vi "CCD1字符识别定位核心转换.vi"(0 "Image In":T1, 1 "ROI Descriptor":T3={"Global Rectangle"=[566, 503, 2033, 1507], "Contours"=[{"ID"=enum."External", "Type"=3, "Coordinates"=[566, 503, 2033, 1507]}]} {"Contours"."Type" items=["No Selection", "Point", "Line", "Rectangle", "Oval", "Polygon", "Freehand Region", "Annulus", "Unused2", "Unused3", "Broken Line", "Freehand Line", "Rotated Rectangle"]}, 2 "Settings":T6={"Curve Parameters"={"Extraction Mode"=0, "Edge Threshold"=35, "Edge Filter Size"=1, "Min Length"=25, "Row Search Step Size"=15, "Col Search Step Size"=15, "Max Endpoint Gap"=10, "Closed"=FALSE, "Subpixel"=FALSE}, "Match Mode"={"Rotation"=TRUE, "Scale"=FALSE, "Occlusion"=TRUE, "Reserved 1"=FALSE, "Reserved 2"=FALSE, "Reserved 3"=FALSE}, "Range Settings"=[{"Match Constraints"=0, "Min"=-17.0, "Max"=17.0}, {"Match Constraints"=2, "Min"=0.0, "Max"=25.0}], "Number of Matches"=1, "Minimum Match Score"=400.0, "SubPixel Accuracy"=FALSE, "Adv. Geometric Match Options 2"=[{"Setup Data Item"=21, "Item Value"=0.0}, {"Setup Data Item"=22, "Item Value"=1.0}]} {"Curve Parameters"."Extraction Mode" items=["Normal", "Uniform Regions"]; "Curve Parameters"."Edge Filter Size" items=["Fine", "Normal", "Contour Tracing"]; "Curve Parameters"."Max Endpoint Gap" min=0; "Curve Parameters"."Col Search Step Size" min=1 max=255 step=1; "Curve Parameters"."Row Search Step Size" min=1 max=255 step=1; "Curve Parameters"."Min Length" min=0; "Curve Parameters"."Edge Threshold" min=1 max=350 step=1; "Range Settings"."Max" format="%.2f"; "Range Settings"."Min" format="%.2f"; "Range Settings"."Match Constraints" items=["Rotation Angle (degrees)", "Scale Factor (%)", "Occlusion (%)"]; "Adv. Geometric Match Options 2"."Setup Data Item" items=["Curve Extraction Mode", "Curve Edge Threshold", "Curve Edge Filter Size", "Min Curve Length", "Curve Row Search Step Size", "Curve Col Search Step Size", "Curve Max Endpoint Gap", "Extract Closed Curves", "Enable Subpixel Curve Extraction", "Enable Correlation Score", "Enable Subpixel Accuracy", "Subpixel Iterations", "Subpixel Tolerance", "Initial Match List Length", "Enable Target Template Curve Score", "Min Match Separation Distance", "Min Match Separation Angle", "Min Match Separation Scale", "Max Match Overlap", "Enable Coarse Result", "Enable Calibration Support", "Enable Contrast Reversal", "Search Strategy", "Refinement Match Factor", "Subpixel Match Factor"]}, 3 "Template File Path":path=path "D:/Inspect System/Source Code/Template Program/字符检测定位模板.png", 6 "Reference System":T2={"Origin"={"X"=1245.2058, "Y"=1038.7815}, "Angle (deg)"=0.021420227, "Axis Reference"=0} {"Axis Reference" items=["Direct", "Indirect"]}, 7 "error in":errorcluster) -> (20 "Image Out":T1, 21 "Matches (Geometric Matching 1)":T8[](array[typedef]) {"Correlation Score" format="%.2f"; "Target Template Curve Score" format="%.2f"; "Template Target Curve Score" format="%.2f"; "Bounding Box"."y" format="%.2f"; "Bounding Box"."x" format="%.2f"; "Position"."y" format="%.2f"; "Position"."x" format="%.2f"; "Score" format="%.2f"; "Scale" format="%.2f"; "Angle" format="%.2f"; "Occlusion %" format="%.2f"}, 22 "Calibrated Matches (Geometric Matching 1)":T8[](array[typedef]) {"Correlation Score" format="%.2f"; "Target Template Curve Score" format="%.2f"; "Template Target Curve Score" format="%.2f"; "Bounding Box"."y" format="%.2f"; "Bounding Box"."x" format="%.2f"; "Position"."y" format="%.2f"; "Position"."x" format="%.2f"; "Score" format="%.2f"; "Scale" format="%.2f"; "Angle" format="%.2f"; "Occlusion %" format="%.2f"}, 23 "Coordinate System Out (Set Coordinate System 1)":T7 {"Measurement System"."Axis Reference" items=["Direct", "Indirect"]; "Measurement System"."Angle (deg)" format="%.2f"; "Measurement System"."Origin"."Y" format="%.2f"; "Measurement System"."Origin"."X" format="%.2f"; "Reference System"."Axis Reference" items=["Direct", "Indirect"]; "Reference System"."Angle (deg)" format="%.2f"; "Reference System"."Origin"."Y" format="%.2f"; "Reference System"."Origin"."X" format="%.2f"}, 24 "Number of Matches (Geometric Matching 1)":i32, 27 "error out":errorcluster)   [LabVIEW 2017]
doc: "Creates, edits, and runs vision algorithms using NI Vision Assistant.\n\nWhen you place this Express VI on the block diagram, NI Vision Assistant launches. Create an algorithm using the Vision Assistant processing functions. After you create an algorithm, you can select the controls and indicators that you want to be able to programmatically set in LabVIEW. Double-click the Vision Assistant Express VI to edit the algorithm."
uses:
  <vilib>/vision/Image Controls.llb/IMAQ Image.ctl
  <vilib>/vision/Pattern Matching.llb/IMAQ GM Match Report.ctl
  <vilib>/vision/Pattern Matching.llb/IMAQ Curve Parameters.ctl
  <vilib>/vision/Pattern Matching.llb/IMAQ Match Range Setting.ctl
  <vilib>/vision/NI_Vision_Development_Module.lvlib
panel:
  out "Image Out 2":T1
  in  "ROI Descriptor 2":T3={"Global Rectangle"=[566, 503, 2033, 1507], "Contours"=[{"ID"=enum."External", "Type"=3, "Coordinates"=[566, 503, 2033, 1507]}]} {"Contours"."Type" items=["No Selection", "Point", "Line", "Rectangle", "Oval", "Polygon", "Freehand Region", "Annulus", "Unused2", "Unused3", "Broken Line", "Freehand Line", "Rotated Rectangle"]}
  # "Range"
types:
  T1 = typedef "IMAQ Image.ctl" = refnum<image>
  T2 = cluster{"Origin":cluster{"X":sgl, "Y":sgl}, "Angle (deg)":sgl, "Axis Reference":u32}
  T3 = cluster{"Global Rectangle":i32[], "Contours":cluster{"ID":enum32{"External", "Internal"}, "Type":u32, "Coordinates":i32[]}[]}
  T4 = typedef "IMAQ Curve Parameters.ctl" = cluster{"Extraction Mode":u32, "Edge Threshold":i32, "Edge Filter Size":u32, "Min Length":i32, "Row Search Step Size":i32, "Col Search Step Size":i32, "Max Endpoint Gap":i32, "Closed":bool, "Subpixel":bool}
  T5 = typedef "IMAQ Match Range Setting.ctl" = cluster{"Match Constraints":u32, "Min":dbl, "Max":dbl}
  T6 = cluster{"Curve Parameters":T4, "Match Mode":cluster{"Rotation":bool, "Scale":bool, "Occlusion":bool, "Reserved 1":bool, "Reserved 2":bool, "Reserved 3":bool}, "Range Settings":T5[], "Number of Matches":i32, "Minimum Match Score":sgl, "SubPixel Accuracy":bool, "Adv. Geometric Match Options 2":cluster{"Setup Data Item":u16, "Item Value":dbl}[]}
  T7 = cluster{"Reference System":cluster{"Origin":cluster{"X":sgl, "Y":sgl}, "Angle (deg)":sgl, "Axis Reference":u32}, "Measurement System":cluster{"Origin":cluster{"X":sgl, "Y":sgl}, "Angle (deg)":sgl, "Axis Reference":u32}}
  T8 = typedef "IMAQ GM Match Report.ctl" = cluster{"Position":cluster{"x":sgl, "y":sgl}, "Angle":sgl, "Scale":sgl, "Score":sgl, "Bounding Box":cluster{"x":sgl, "y":sgl}[], "Contrast Reversed":bool, "Occlusion %":sgl, "Template Target Curve Score":sgl, "Target Template Curve Score":sgl, "Correlation Score":sgl}
  T9 = enum16{"Reset", "Update Coordinate System", "Get Coordinate System"}
  T10 = enum16{"Horizontal Motion", "Vertical Motion", "Horizontal and Vertical Motion", "Horizontal, Vertical and Angular Motion"}
  T11 = cluster{"Number of Matches Requested":i32, "Minimum Match Score":sgl, "Angle Ranges":cluster{"Start Angle":sgl, "End Angle":sgl}[]}
  T12 = cluster{"Position":cluster{"x":sgl, "y":sgl}, "Angle":sgl, "Scale":sgl, "Score":sgl, "Bounding Box":cluster{"x":sgl, "y":sgl}[]}[]
  T13 = typedef "IMAQ Coordinate System" = cluster{"Reference System":cluster{"Origin":cluster{"X":sgl, "Y":sgl}, "Angle (deg)":sgl, "Axis Reference":u32}, "Measurement System":cluster{"Origin":cluster{"X":sgl, "Y":sgl}, "Angle (deg)":sgl, "Axis Reference":u32}}
  T14 = typedef "Image Type" = u32
  T15 = cluster{"Backup Image Name":string, "Coordinate System Out":T13}
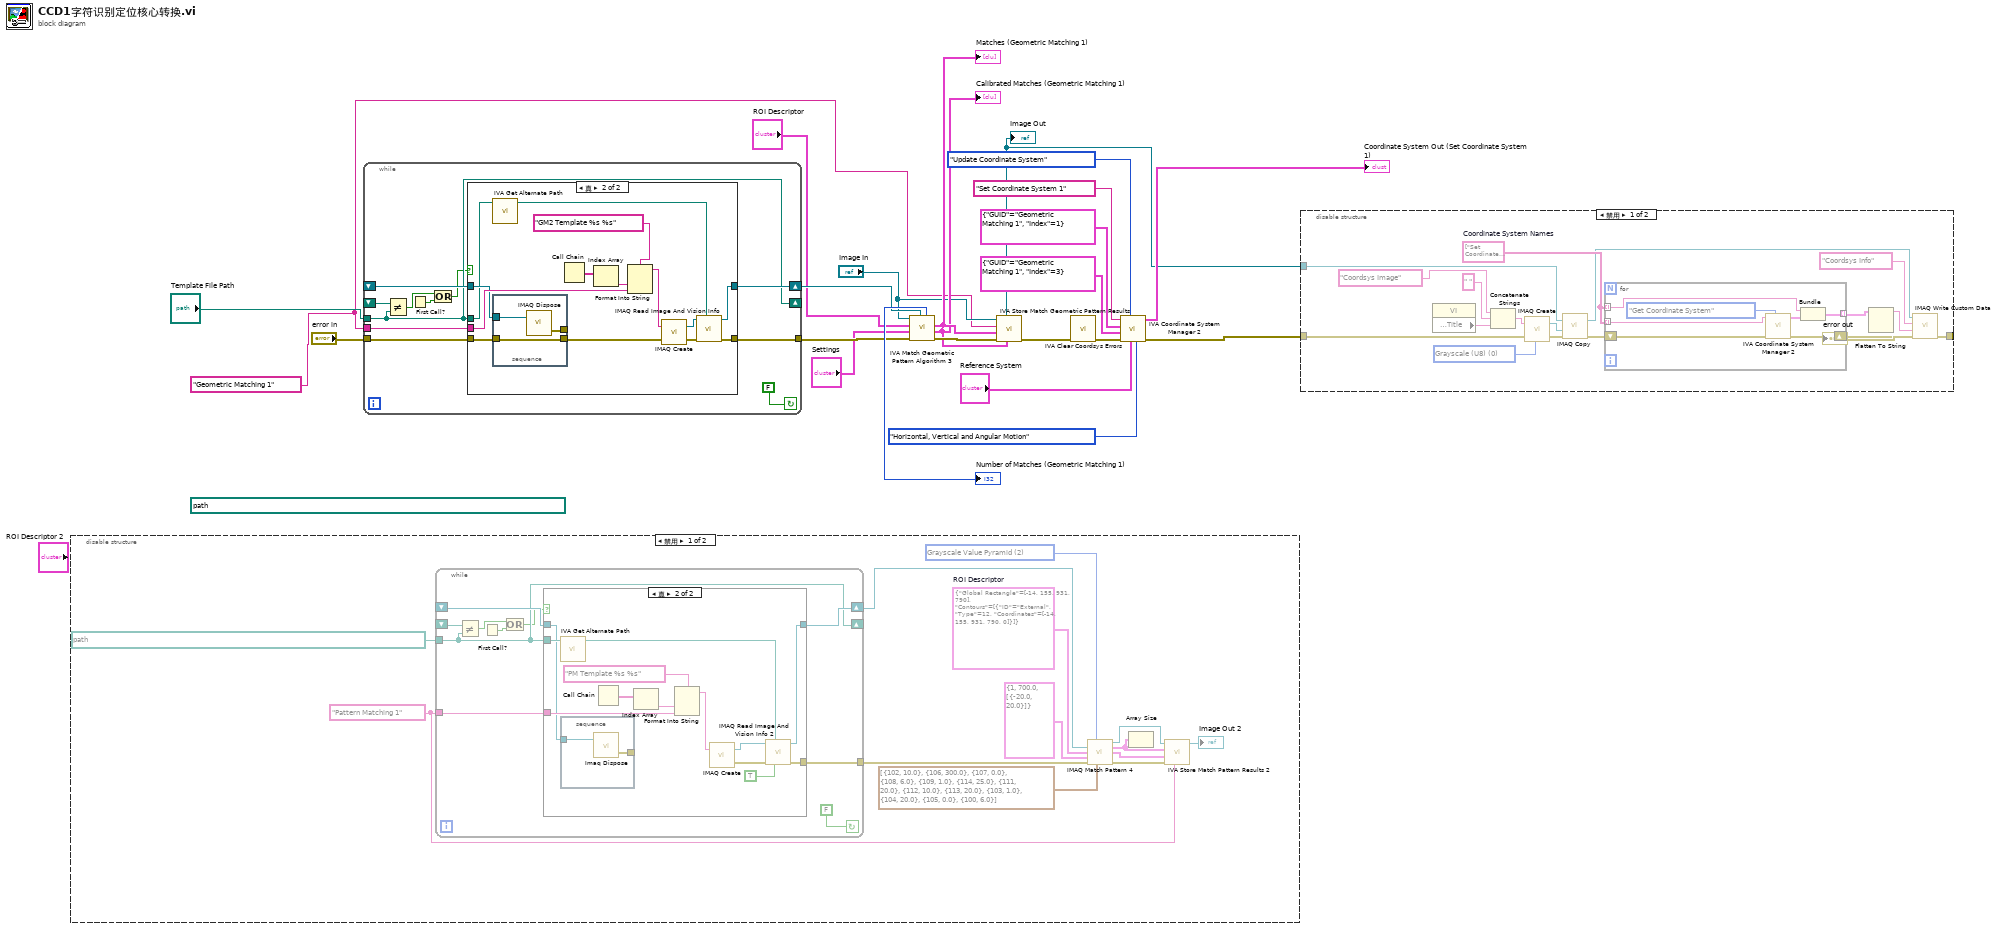
[diagram p0: block diagram]
diagram:
  w1 = "Geometric Matching 1" ("Step Name")
  (unwired) path "F:/Inspect System -2/Source Code/Template Program/程序1/字符定位模板.png" ("Template File Path")
  n1 = disable-structure shown="禁用" {
    frame Disabled {
      w34 = 2 items=["All", "Low Discrepancy Sampling", "Grayscale Value Pyramid", "Gradients Pyramid"] ("Algorithm")
      w31 = "Pattern Matching 1" ("Step Name")
      w33 = T3 {"Global Rectangle"=[-14, 155, 931, 790], "Contours"=[{"ID"=enum."External", "Type"=12, "Coordinates"=[-14, 155, 931, 790, 0]}]}  # ROI Descriptor
      n2 = while {
        shift-right: [w47] -> w28
        shift-left: _ -> [w46]
        tunnel: [w44] -> w27
        tunnel: path "D:/Inspect System/Source Code/Template Program/字符检测定位模板.png" ("Template File Path") -> [w41]
        tunnel: w31 -> [w43]
        shift-right: [w41] -> _
        shift-left: _ -> [w42]
        stop <- FALSE continue-if-true
        n3 = Not Equal?(x=w42, y=w41) -> (x != y?=w39:bool)
        n4 = First Call?() -> (First Call?: T/F=w40:bool)
        n5 = Or(x=w39, y=w40) -> (x .or. y?=w38:bool)
        n6 = case "条件结构" shown="真" w38 {
          tunnel: [w48 w52] -> w47
          tunnel: w46 -> [w48 w55]
          tunnel: [_ w53] -> w44
          tunnel: w41 -> [_ w56]
          tunnel: w43 -> [_ w57]
          frame False {
          }
          frame True {
            n7 = call <vilib>:"IVA Get Alternate Path.vi"("Path In"=w56) -> ("Path Out"=w54:path)  [unwired: 10 out]
            n8 = stacked-sequence "层叠式顺序结构" {
              tunnel: w55 -> [w63]
              tunnel: [w62] -> _
              frame #0 {
                n9 = call "Imaq Dispose"("Image"=w63) -> ("error out"=w62:errorcluster)  [unwired: 2 in, 3 out]
              }
            }
            n10 = Call Chain() -> (call chain=w59:string[])
            n11 = Index Array(array=w59) -> (element=w58:string)  [unwired: 1 in]
            n12 = Format Into String(format string="PM Template %s %s" ("Image Name"), w58, w57) -> (resulting string=w61:string)  [unwired: 2 in, 1 out]
            n13 = call "IMAQ Create"("Image Name"=w61) -> ("New Image"=w51:T1, "error out"=w50:errorcluster)  [unwired: 3 in, 1 out]
            n14 = call "IMAQ Read Image And Vision Info 2"("Use File Path Image Type"=TRUE, "File Path"=w54, "error in (no error)"=w50, "Image"=w51) -> ("error out"=w53:errorcluster, "Image Out"=w52:T1)  [unwired: 5 in, 1 out]
          }
        }
      }
      n15 = call "IMAQ Match Pattern 4"("Algorithm"=w34, "Template Image"=w28, "ROI Descriptor"=w33, "Parameters"=T11 {"Number of Matches Requested"=1, "Minimum Match Score"=700.0, "Angle Ranges"=[{"Start Angle"=-20.0, "End Angle"=20.0}]}, "error in (no error)"=w27, "Advanced Options"=cluster{"Item":u16, "Value":dbl}[] [{"Item"=102, "Value"=10.0}, {"Item"=106, "Value"=300.0}, {"Item"=107, "Value"=0.0}, {"Item"=108, "Value"=6.0}, {"Item"=109, "Value"=1.0}, {"Item"=114, "Value"=25.0}, {"Item"=111, "Value"=20.0}, {"Item"=112, "Value"=10.0}, {"Item"=113, "Value"=20.0}, {"Item"=103, "Value"=1.0}, {"Item"=104, "Value"=20.0}, {"Item"=105, "Value"=0.0}, {"Item"=100, "Value"=6.0}]) -> ("Image (duplicate)"=w35:T1, "Matches (pixel)"=w30:T12, "Matches (real-world)"=w29:T12, "error out"=w36:errorcluster)  [unwired: 5 in, 1 out]
      n16 = Array Size(array=w30) -> ()  [unwired: 1 out]
      n17 = call <vilib>:"IVA Store Match Pattern Results 2.vi"("Step Name"=w31, "error in (no error)"=w36, "Matches (real-world)"=w29, "Matches (pixel)"=w30, "Image in"=w35) -> ("Image dup"=→"Image Out 2":T1)  [unwired: 1 in, 5 out]
    }
    frame Enabled {
    }
  }
  n18 = while {
    shift-right: [w74] -> w18
    shift-left: _ -> [w73]
    tunnel: [w71] -> w19
    tunnel: "error in" -> [w70]
    tunnel: "Template File Path" -> [w67]
    tunnel: w1 -> [w69]
    shift-right: [w67] -> _
    shift-left: _ -> [w68]
    stop <- FALSE continue-if-true
    n19 = Not Equal?(x=w68, y=w67) -> (x != y?=w65:bool)
    n20 = First Call?() -> (First Call?: T/F=w66:bool)
    n21 = Or(x=w65, y=w66) -> (x .or. y?=w64:bool)
    n22 = case "条件结构" shown="真" w64 {
      tunnel: [w76 w89] -> w74
      tunnel: w73 -> [w76 w81]
      tunnel: [w75 w86] -> w71
      tunnel: w70 -> [w75 w82]
      tunnel: w69 -> [_ w83]
      tunnel: w67 -> [_ w80]
      frame False {
      }
      frame True {
        n23 = call <vilib>:"IVA Get Alternate Path.vi"("Path In"=w80) -> ("Path Out"=w79:path)  [unwired: 10 out]
        n24 = stacked-sequence "层叠式顺序结构" {
          tunnel: w82 -> [w93]
          tunnel: w81 -> [w92]
          tunnel: [w93] -> w78
          tunnel: [w91] -> _
          frame #0 {
            n25 = call "IMAQ Dispose"("Image"=w92) -> ("error out"=w91:errorcluster)  [unwired: 2 in, 3 out]
          }
        }
        n26 = Call Chain() -> (call chain=w85:string[])
        n27 = Index Array(array=w85) -> (element=w84:string)  [unwired: 1 in]
        n28 = Format Into String(format string="GM2 Template %s %s" ("Image Name"), w84, w83) -> (resulting string=w90:string)  [unwired: 2 in, 1 out]
        n29 = call "IMAQ Create"("Image Name"=w90, "error in (no error)"=w78) -> ("New Image"=w88:T1, "error out"=w87:errorcluster)  [unwired: 2 in, 1 out]
        n30 = call "IMAQ Read Image And Vision Info"("File Path"=w79, "error in (no error)"=w87, "Image"=w88) -> ("error out"=w86:errorcluster, "Image Out"=w89:T1)  [unwired: 1 in, 6 out]
      }
    }
  }
  n31 = call <vilib>:"IVA Match Geometric Pattern Algorithm 3.vi"("Template"=w18, "error in (no error)"=w19, "Settings"="Settings", "ROI Descriptor"="ROI Descriptor", "Image"="Image In") -> ("error out"=w23:errorcluster, "Calibrated Matches"=w21:T8[], "Matches"=w22:T8[], "Number of Matches"=→"Number of Matches (Geometric Matching 1)":i32)  [unwired: 3 out]
  "Matches (Geometric Matching 1)" <- w22
  "Calibrated Matches (Geometric Matching 1)" <- w21
  n32 = call <vilib>:"IVA Store Match Geometric Pattern Results.vi"("Calibrated Matches"=w21, "error in (no error)"=w23, "Matches"=w22, "Step Name"=w1, "Image in"="Image In") -> ("error out"=w17:errorcluster, "Image dup"=w6:T1)  [unwired: 5 out]
  "Image Out" <- w6
  n33 = call <vilib>:"IVA Clear Coordsys Errors.vi"("error in (no error)"=w17) -> ("error out"=w16:errorcluster)  [unwired: 10 in]
  n34 = call <vilib>:"IVA Coordinate System Manager 2.vi"("Mode"=T10."Horizontal, Vertical and Angular Motion", "Reference System"="Reference System", "Function"=T9."Update Coordinate System", "error in (no error)"=w16, "Angle ID"=cluster{"GUID":string, "Index":i32} {"GUID"="Geometric Matching 1", "Index"=3}, "Origin ID"=cluster{"GUID":string, "Index":i32} {"GUID"="Geometric Matching 1", "Index"=1}, "Coordinate System Name"="Set Coordinate System 1") -> ("error out"=w9:errorcluster, "Coordinate System Out"=→"Coordinate System Out (Set Coordinate System 1)":T13)  [unwired: 3 out]
  n35 = disable-structure shown="禁用" {
    disable-tunnel: w9 -> [w110 w118]
    disable-tunnel: [w100 w118] -> w7
    disable-tunnel: w6 -> [w94 _]
    frame Disabled {
      w97 = T14 0 items=["Grayscale (U8)", "Grayscale (I16)", "Grayscale (SGL)", "Complex (CSG)", "RGB (U32)", "HSL (U32)", "RGB (U64)", "Grayscale (U16)"] ("Image Type")
      w104 = string[] ["Set Coordinate System 1"]  # Coordinate System Names
      n36 = property class="VI"() -> ("Front Panel Window:Title"=w98:string)  [unwired: 2 in, 2 out]
      n37 = Concatenate Strings("Coordsys Image" ("Processed Image Name"), " ", w98) -> (w107:string)
      n38 = call "IMAQ Create"("Image Name"=w107, "Image Type"=w97, "error in (no error)"=w110) -> ("New Image"=w105:T1, "error out"=w106:errorcluster)  [unwired: 1 in, 1 out]
      n39 = call "IMAQ Copy"("error in (no error)"=w106, "Image Dst"=w105, "Image Src"=w94) -> ("error out"=w96:errorcluster, "Image Dst Out"=w103:T1)  [unwired: 3 out]
      n40 = for "For循环" {
        tunnel: w104 -> [w116] mode=indexing
        tunnel: w104 -> [w114] mode=indexing
        tunnel: [w113] -> w102 mode=indexing
        shift-right: [w111] -> w95
        shift-left: w96 -> [w112]
        n41 = call <vilib>:"IVA Coordinate System Manager 2.vi"("Function"=T9."Get Coordinate System", "error in (no error)"=w112, "Coordinate System Name"=w116) -> ("error out"=w111:errorcluster, "Coordinate System Out"=w115:T13)  [unwired: 4 in, 3 out]
        n42 = Bundle("Backup Image Name"=w114, "Coordinate System Out"=w115) -> (w113:T15)  [unwired: 1 out]
      }
      n43 = Flatten To String(anything=w102) -> (data string=w101:string)  [unwired: 1 in, 4 out]
      n44 = call "IMAQ Write Custom Data"("error in (no error)"=w95, "Custom Data In"=w101, "Key"="Coordsys Info", "Image"=w103) -> ("error out"=w100:errorcluster)  [unwired: 7 out]
    }
    frame Enabled {
    }
  }
  "error out" <- w7
